vi "Initialize Image.vi"(8 "error in (no error)":errorcluster, 11 "data type":T2) -> (0 "error out":errorcluster, 2 "Gray Image Out":T1, 3 "Color Image Out":T1)   [LabVIEW 2025, in "Automotive Vision.lvclass"]
uses:
  <instrlib>/FlexRIO/CSI-2/v2/Common/Types/LLP Data Type.ctl
  <vilib>/vision/Image Controls.llb/IMAQ Image.ctl
  Automotive Vision.lvclass
  Automotive Vision.lvclass/Automotive Vision.ctl
  <instrlib>/FlexRIO/CSI-2/v2/Common/NI CSI-2 API Common v2.lvlib
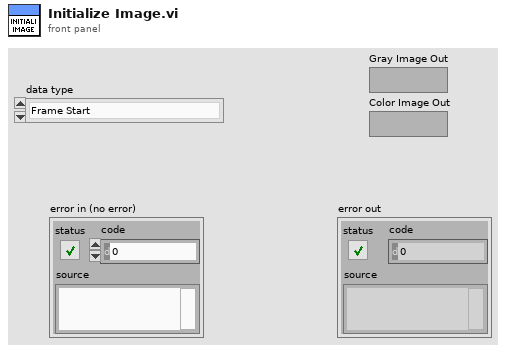
[diagram p1: front panel]
types:
  T1 = typedef "IMAQ Image.ctl" = refnum<image>
  T2 = typedef "NI CSI-2 API Common v2.lvlib/LLP Data Type.ctl" = enum8{"Frame Start", "Frame End", "Line Start", "Line End", "End of Transmission", "Reserved 0", "Reserved 1", "Reserved 2", "Generic Short Packet 1", "Generic Short Packet 2", "Generic Short Packet 3", "Generic Short Packet 4", "Generic Short Packet 5", "Generic Short Packet 6", "Generic Short Packet 7", "Generic Short Packet 8", "Null", "Blanking Data", "Embedded 8-bit non Image Data", "Generic Long Packet 1", "Generic Long Packet 2", "Generic Long Packet 3", "Generic Long Packet 4", "Reserved 3", "YUV420 8-bit", "YUV420 10-bit", "Legacy YUV420 8-bit", "Reserved 4", "YUV420 8-bit Chroma Shifted", "YUV420 10-bit Chroma Shifted", "YUV422 8-bit", "YUV422 10-bit", "RGB444", "RGB555", "RGB565", "RGB666", "RGB888", "Reserved 5", "Reserved 6", "RAW 24", "RAW 6", "RAW 7", "RAW 8", "RAW 10", "RAW 12", "RAW 14", "RAW 16", "RAW 20", "User Defined 8-bit Data 1", "User Defined 8-bit Data 2", "User Defined 8-bit Data 3", "User Defined 8-bit Data 4", "User Defined 8-bit Data 5", "User Defined 8-bit Data 6", "User Defined 8-bit Data 7", "User Defined 8-bit Data 8", "USL Command", "Reserved 7", "Reserved 8", "Reserved 9", "Reserved 10", "Reserved 11", "Reserved 12", "LRTE EPD Spacer"}
  T3 = typedef "Image Type" = u32
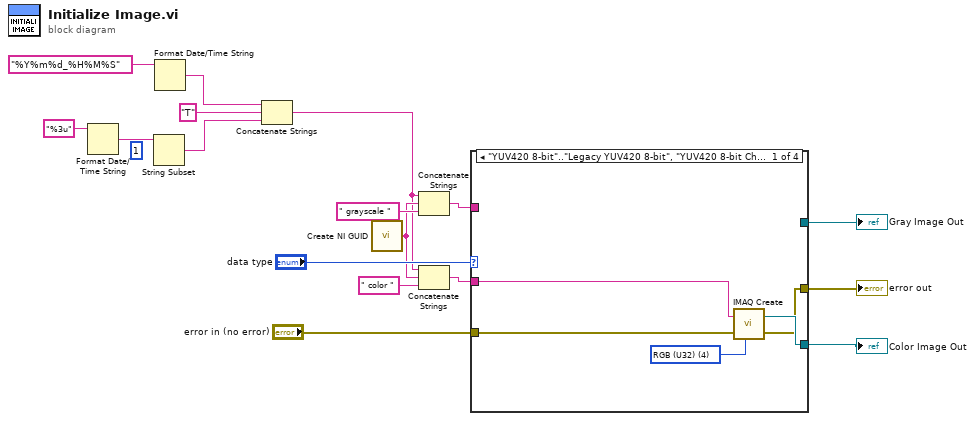
[diagram p0: block diagram]
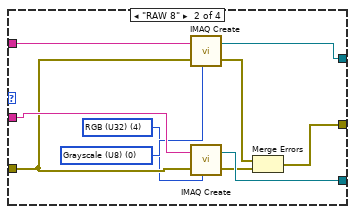
[diagram p2: hidden frame]
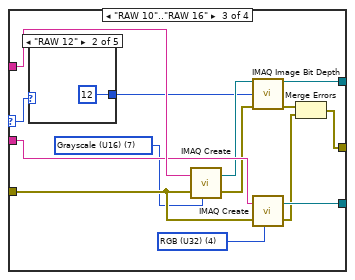
[diagram p3: hidden frame]
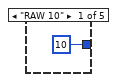
[diagram p4: hidden frame]
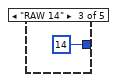
[diagram p5: hidden frame]
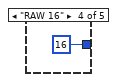
[diagram p6: hidden frame]
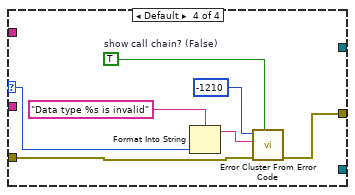
[diagram p8: hidden frame]
diagram:
  (unwired) 1 ("offset (0)")
  n1 = Format Date/Time String(time format string (%c)="%3u") -> (date/time string=w4:string)  [unwired: 2 in]
  n2 = String Subset(string=w4) -> (substring=w2:string)  [unwired: 2 in]
  n3 = Format Date/Time String(time format string (%c)="%Y%m%d_%H%M%S") -> (date/time string=w5:string)  [unwired: 2 in]
  n4 = Concatenate Strings(w5, "T" ("string"), w2) -> (w1:string)
  n5 = call <vilib>:"Create NI GUID.vi"() -> ("NI GUID"=w13:string)
  n6 = Concatenate Strings(w1, w13, " grayscale " ("Image Name")) -> (w16:string)
  n7 = Concatenate Strings(w1, w13, " color " ("Image Name")) -> (w15:string)
  n8 = case shown="\"YUV420 8-bit\"..\"Legacy YUV420 8-bit\", \"YUV420 8-bit Chroma Shifted\"..\"YUV422 10-bit\", \"RGB565\"..\"RGB888\"" "data type" {
    selector: "data type" -> [_ _ w40 w54]
    tunnel: w16 -> [_ w32 w46 _]
    tunnel: w15 -> [w21 w31 w45 _]
    tunnel: "error in (no error)" -> [w20 w30 w44 w52]
    tunnel: [w18 w29 w43 w51] -> w8
    tunnel: [w19 w28 w42 _] -> w9
    tunnel: [_ w27 w41 _] -> w10
    frame "YUV420 8-bit".."Legacy YUV420 8-bit", "YUV420 8-bit Chroma Shifted".."YUV422 10-bit", "RGB565".."RGB888" {
      w22 = T3 4 items=["Grayscale (U8)", "Grayscale (I16)", "Grayscale (SGL)", "Complex (CSG)", "RGB (U32)", "HSL (U32)", "RGB (U64)", "Grayscale (U16)"] ("Image Type")
      n9 = call "IMAQ Create"("Image Name"=w21, "Image Type"=w22, "error in (no error)"=w20) -> ("New Image"=w19:T1, "error out"=w18:errorcluster)  [unwired: 2 in]
    }
    frame "RAW 8" {
      w25 = T3 4 items=["Grayscale (U8)", "Grayscale (I16)", "Grayscale (SGL)", "Complex (CSG)", "RGB (U32)", "HSL (U32)", "RGB (U64)", "Grayscale (U16)"] ("Image Type")
      w26 = T3 0 items=["Grayscale (U8)", "Grayscale (I16)", "Grayscale (SGL)", "Complex (CSG)", "RGB (U32)", "HSL (U32)", "RGB (U64)", "Grayscale (U16)"] ("Image Type")
      n10 = call "IMAQ Create"("Image Name"=w32, "Image Type"=w26, "error in (no error)"=w30) -> ("New Image"=w27:T1, "error out"=w23:errorcluster)  [unwired: 2 in]
      n11 = call "IMAQ Create"("Image Name"=w31, "Image Type"=w25, "error in (no error)"=w30) -> ("New Image"=w28:T1, "error out"=w24:errorcluster)  [unwired: 2 in]
      n12 = Merge Errors(w23, w24) -> (w29:errorcluster)
    }
    frame "RAW 10".."RAW 16" {
      w38 = T3 4 items=["Grayscale (U8)", "Grayscale (I16)", "Grayscale (SGL)", "Complex (CSG)", "RGB (U32)", "HSL (U32)", "RGB (U64)", "Grayscale (U16)"] ("Image Type")
      w39 = T3 7 items=["Grayscale (U8)", "Grayscale (I16)", "Grayscale (SGL)", "Complex (CSG)", "RGB (U32)", "HSL (U32)", "RGB (U64)", "Grayscale (U16)"] ("Image Type")
      n13 = case shown="\"RAW 12\"" w40 {
        tunnel: [u32 10 ("Bit Depth (0)") u32 12 ("Bit Depth (0)") u32 14 ("Bit Depth (0)") u32 16 ("Bit Depth (0)") _] -> w33
        frame "RAW 10" {
        }
        frame "RAW 12" {
        }
        frame "RAW 14" {
        }
        frame "RAW 16" {
        }
        frame Default {
        }
      }
      n14 = call "IMAQ Create"("Image Name"=w46, "Image Type"=w39, "error in (no error)"=w44) -> ("New Image"=w36:T1, "error out"=w35:errorcluster)  [unwired: 2 in]
      n15 = call "IMAQ Image Bit Depth"("Image"=w36, "Bit Depth (0)"=w33, "error in (no error)"=w35) -> ("Image Out"=w41:T1, "error out"=w34:errorcluster)  [unwired: 10 in, 1 out]
      n16 = call "IMAQ Create"("Image Name"=w45, "Image Type"=w38, "error in (no error)"=w44) -> ("New Image"=w42:T1, "error out"=w37:errorcluster)  [unwired: 2 in]
      n17 = Merge Errors(w34, w37) -> (w43:errorcluster)
    }
    frame Default {
      w56 = TRUE  # show call chain? (False)
      n18 = Format Into String(format string="Data type %s is invalid" ("error message (\"\")"), w54) -> (resulting string=w53:string)  [unwired: 2 in, 1 out]
      n19 = call <vilib>:"Error Cluster From Error Code.vi"("show call chain? (False)"=w56, "error in (no error)"=w52, "error message (\"\")"=w53, "error code (0)"=-1210) -> ("error out"=w51:errorcluster)  [unwired: 5 in]
    }
  }
  "Gray Image Out" <- w10
  "Color Image Out" <- w9
  "error out" <- w8
